vi "Destroy Listen Events.vi"(8 "error in (no error)":errorcluster, 11 "CIFCorePlugin in":refnum<class "CIFCorePlugin.lvclass">) -> (0 "error out":errorcluster, 3 "CIFCorePlugin out":refnum<class "CIFCorePlugin.lvclass">)   [LabVIEW 2021, in "CIFCorePlugin.lvclass"]
uses:
  CIFCorePlugin.lvclass
  Typedef/Listen Events.ctl
  CIFCorePlugin.lvclass/CIFCorePlugin.ctl
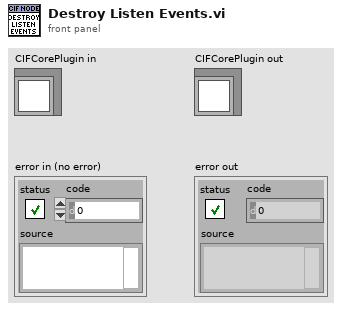
[diagram p1: front panel]
types:
  T1 = typedef "CIFCorePlugin.lvclass/Listen Events.ctl" = cluster{"Comm":refnum<user-event>, "Prepare":refnum<user-event>, "Execute":refnum<user-event>, "Pause":refnum<user-event>, "Destroy":refnum<user-event>}
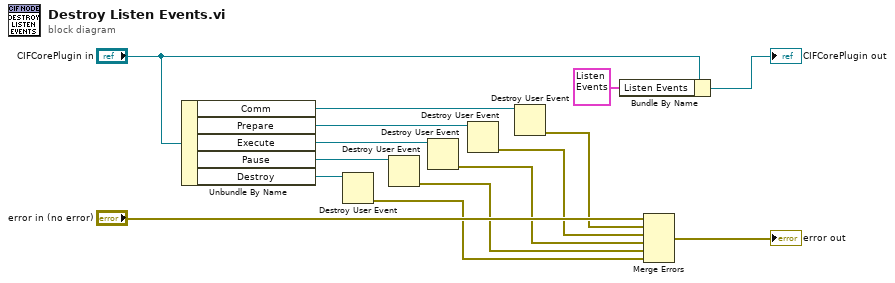
[diagram p0: block diagram]
diagram:
  n1 = Unbundle By Name("CIFCorePlugin in") -> ("Comm"=w9:refnum<user-event>, "Prepare"=w5:refnum<user-event>, "Execute"=w6:refnum<user-event>, "Pause"=w7:refnum<user-event>, "Destroy"=w8:refnum<user-event>)
  n2 = Destroy User Event(user event=w8) -> (error out=w1:errorcluster)  [unwired: 1 in]
  n3 = Destroy User Event(user event=w7) -> (error out=w2:errorcluster)  [unwired: 1 in]
  n4 = Destroy User Event(user event=w6) -> (error out=w3:errorcluster)  [unwired: 1 in]
  n5 = Destroy User Event(user event=w5) -> (error out=w4:errorcluster)  [unwired: 1 in]
  n6 = Destroy User Event(user event=w9) -> (error out=w11:errorcluster)  [unwired: 1 in]
  n7 = Bundle By Name(cluster="CIFCorePlugin in", "Listen Events"=T1 {"Comm"=refnum, "Prepare"=refnum, "Execute"=refnum, "Pause"=refnum, "Destroy"=refnum}) -> (→"CIFCorePlugin out":refnum<class "CIFCorePlugin.lvclass">)
  n8 = Merge Errors("error in (no error)", w11, w4, w3, w2, w1) -> (→"error out":errorcluster)
